vi "Read settings.vi"(8 "error in (no error)":errorcluster, 11 "Analog_Input in":refnum<class "Analog_Input.lvclass">) -> (0 "error out":errorcluster, 2 "settings":T1={"enable"=FALSE, "samples_per_measurement"=1, "sample rate (Hz)"=-10.0, "source"="Dev3/ai0:2", "Start Trigger"={"Wait for start trigger?"=FALSE, "source"="/Dev1/PFI0", "edge"=10280}} {"Start Trigger"."edge" items=["Rising"=10280, "Falling"=10171]}, 3 "Analog_Input out":refnum<class "Analog_Input.lvclass">)   [LabVIEW 2013, in "Analog_Input.lvclass"]
uses:
  Analog_Input.lvclass
  settings.ctl
  Analog_Input.lvclass/Analog_Input.ctl
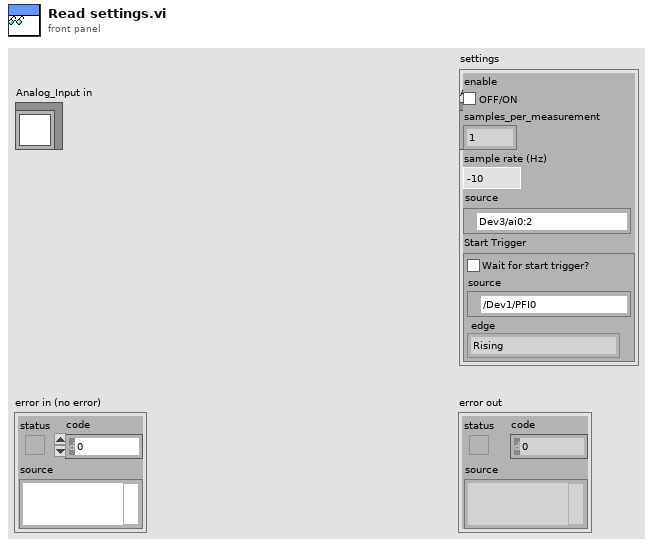
[diagram p1: front panel]
types:
  T1 = typedef "Analog_Input.lvclass/settings.ctl" = cluster{"enable":bool, "samples_per_measurement":i32, "sample rate (Hz)":dbl, "source":tag, "Start Trigger":cluster{"Wait for start trigger?":bool, "source":tag, "edge":i32}}
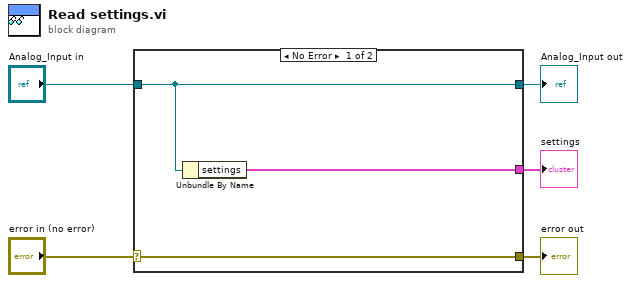
[diagram p0: block diagram]
diagram:
  n1 = case shown="No Error" "error in (no error)" {
    selector: "error in (no error)" -> [w8 w9]
    tunnel: [w8 w9] -> w4
    tunnel: [w7 w10] -> w2
    tunnel: "Analog_Input in" -> [w7 w10]
    tunnel: [w6 _] -> w1
    frame No Error {
      n2 = Unbundle By Name(w7) -> ("settings"=w6:T1)
    }
    frame Error {
    }
  }
  "error out" <- w4
  "Analog_Input out" <- w2
  "settings" <- w1
